vi "labviewharkka.vi"() -> ()   [LabVIEW 2018]
uses:
  <vilib>/platform/TimedLoop/XDataNode/XDataNode.xnode
  <vilib>/Platform/TimedLoop/XDataNode/nitl_modes.ctl
  <vilib>/Platform/TimedLoop/XDataNode/XDNodeRunTimeDep.lvlib
  <vilib>/Platform/TimedLoop/XDataNode/wakeup.ctl
  <vilib>/Platform/TimedLoop/XDataNode/timing_clust.ctl
panel:
  in  "stop":bool
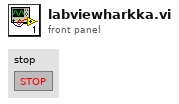
[diagram p1: front panel]
types:
  T1 = typedef "XDNodeRunTimeDep.lvlib/timing_clust.ctl" = cluster{"Expected End [f-1]":u64, "Actual End [f-1]":u64, "Finished Late? [f-1]":bool, "Expected End [i-1]":u64, "Actual End [i-1]":u64, "Finished Late? [i-1]":bool, "Expected Start [i]":u64, "Actual Start [i]":u64, "Expected Start [f]":u64, "Actual Start [f]":u64, "Source Name":string, "Structure Name":string, "Period":i64, "Deadline":i64, "Offset":i64, "Start":i64, "Priority":i32, "Timeout":i32, "Mode":T2, "Wakeup Reason":T3, "Error":errorcluster, "Source Type":string, "Secondary Source Type":string, "Global End Time":u64, "Global Start Time":u64, "Frame Duration":u64, "Iteration Duration":u64, "Assigned CPU":i32, "I/O Scan Engine Mode":u32}
  T2 = typedef "XDNodeRunTimeDep.lvlib/nitl_modes.ctl" = enum32{"No Change", "Process missed periods, maintain original phase", "Discard missed periods, maintain original phase", "Process missed periods, ignore original phase", "Discard missed periods, ignore original phase"}
  T3 = typedef "XDNodeRunTimeDep.lvlib/wakeup.ctl" = enum32{"Normal", "Aborted", "Asynchronous wakeup", "Timing source error", "Timed loop error", "Timeout"}
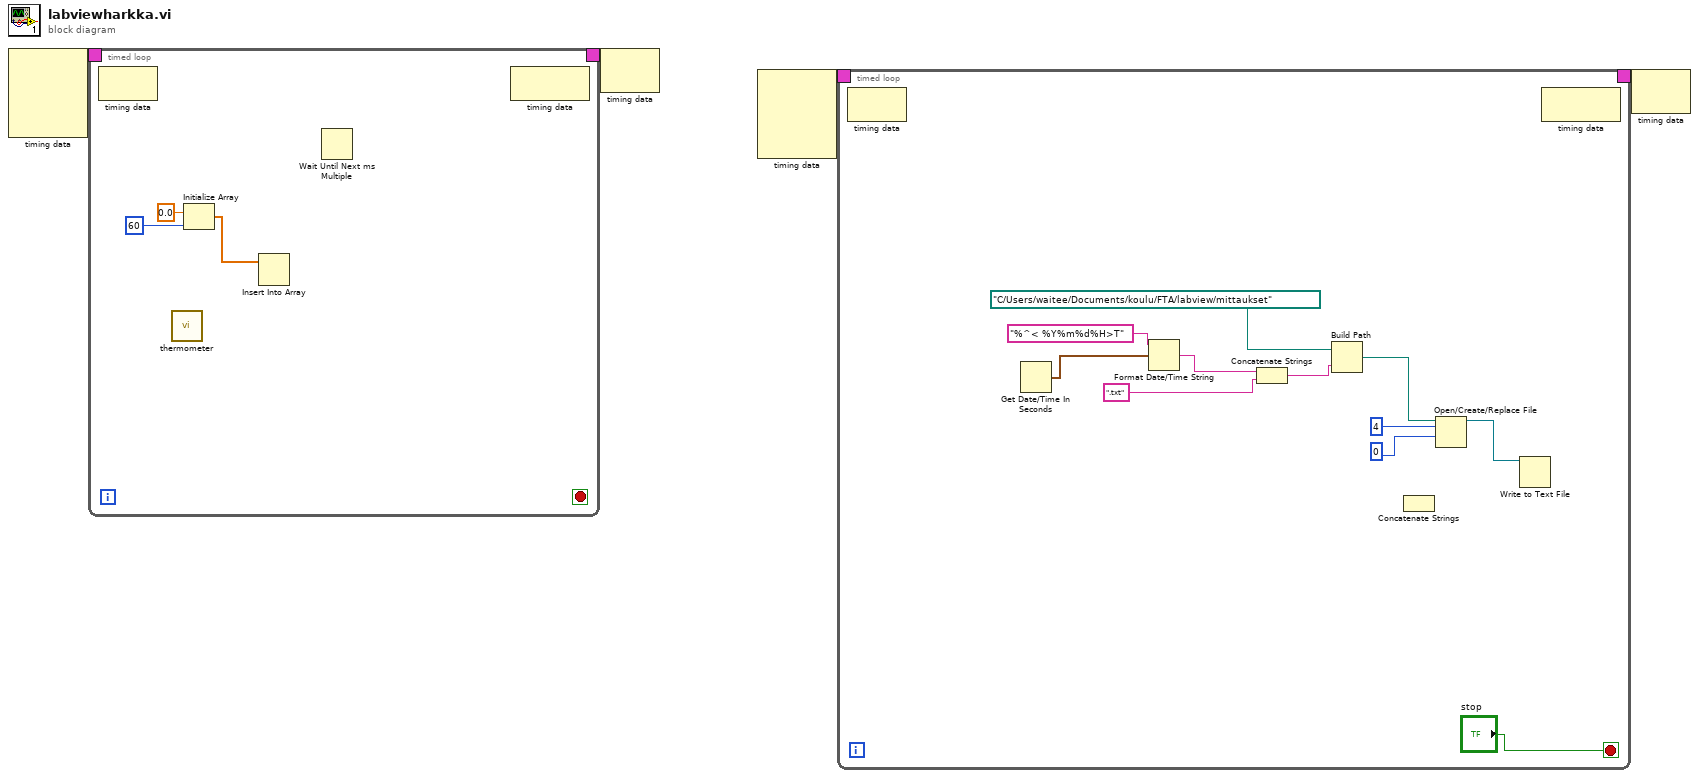
[diagram p0: block diagram]
diagram:
  n1 = node-c288() -> (w4:T1)  [unwired: 4 in]
  n2 = timed-loop {
    timing: w4 -> [_]
    timing-out: [_] -> w3
    stop <- _ stop-if-true
    n3 = node-c288() -> ()  [unwired: 1 in, 1 out]
    n4 = call "thermometer.vi"() -> ()  [unwired: 1 in, 1 out]
    n5 = Initialize Array(0.0 ("element"), 60 ("dimension size")) -> (w5:dbl[])
    n6 = Insert Into Array(array=w5) -> ()  [unwired: 2 in, 1 out]
    n7 = Wait Until Next ms Multiple() -> ()  [unwired: 1 in, 1 out]
    n8 = node-c288() -> ()  [unwired: 1 in, 1 out]
  }
  n9 = node-c288(w3) -> ()  [unwired: 1 out]
  n10 = node-c288() -> (w2:T1)  [unwired: 4 in]
  n11 = timed-loop {
    timing: w2 -> [_]
    timing-out: [_] -> w1
    stop <- "stop" stop-if-true
    n12 = node-c288() -> ()  [unwired: 1 in, 1 out]
    n13 = Get Date/Time In Seconds() -> (seconds since 1Jan1904=w12:timestamp)
    n14 = Format Date/Time String(time format string (%c)="%^< %Y%m%d%H>T", seconds (now)=w12) -> (date/time string=w18:string)  [unwired: 1 in]
    n15 = Concatenate Strings(w18, ".txt") -> (w16:string)
    n16 = Build Path(base path=path "C:/Users/waitee/Documents/koulu/FTA/labview/mittaukset", name or relative path=w16) -> (appended path=w14:path)
    n17 = Concatenate Strings() -> ()  [unwired: 2 in, 1 out]
    n18 = Open/Create/Replace File(file path (use dialog)=w14, operation (0:open)=4, access (0:read/write)=0) -> (refnum out=w11:refnum<file>)  [unwired: 3 in, 2 out]
    n19 = Write to Text File(file (use dialog)=w11) -> ()  [unwired: 3 in, 3 out]
    n20 = node-c288() -> ()  [unwired: 1 in, 1 out]
  }
  n21 = node-c288(w1) -> ()  [unwired: 1 out]
